vi "Image Display Loop.vi"(0 "fpga interface in":refnum<k20>, 1 "'stop' notifier":refnum<notifier>, 2 "rate references":T1(array[cluster]), 5 "raw display notifier":refnum<notifier>, 7 "display references":refnum<vi>[](array[refnum]), 11 "error in (no error)":errorcluster) -> (15 "error out":errorcluster)   [LabVIEW 2023, in "GettingStarted_Common_148X_Host.lvlib"]
uses:
  GettingStarted_Common_148X_Host.lvlib
  <vilib>/vision/Image Controls.llb/IMAQ Image.ctl
  Types/Serial Channel Display Parameters.ctl
  Types/RAW Interpretation for Display.ctl
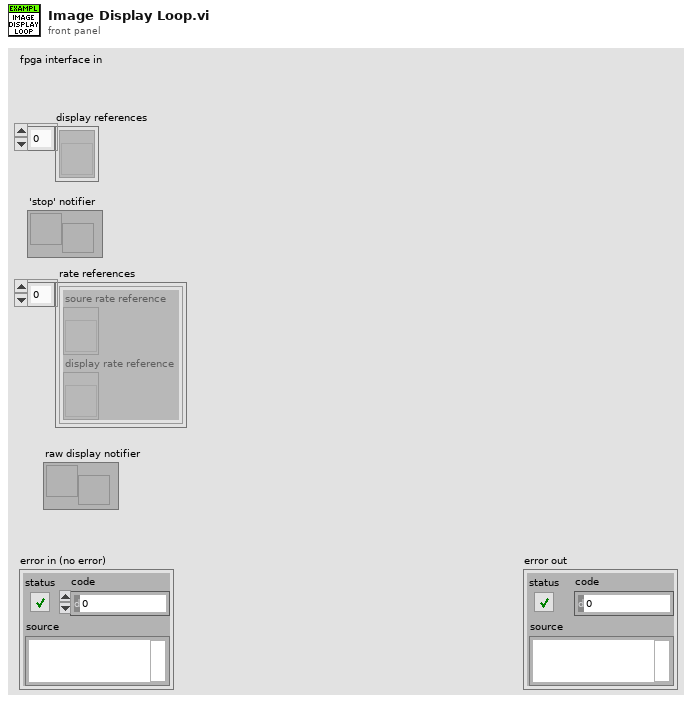
[diagram p1: front panel]
types:
  T1 = cluster{"soure rate reference":refnum<vi>, "display rate reference":refnum<vi>}[]
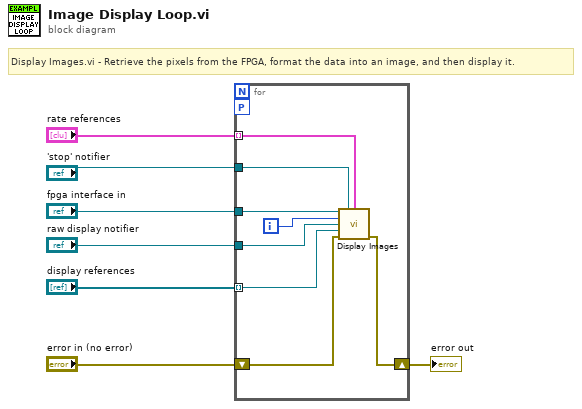
[diagram p0: block diagram]
diagram:
  # "Display Images.vi - Retrieve the pixels from the FPGA, format the data into an image, and then display it."
  n1 = for {
    tunnel: "fpga interface in" -> [w15]
    shift-right: [w12] -> w6
    shift-left: "error in (no error)" -> [w13]
    tunnel: "display references" -> [w14] mode=indexing
    tunnel: "rate references" -> [w10] mode=indexing
    workers-P: _ -> [_]
    tunnel: "'stop' notifier" -> [w9]
    tunnel: "raw display notifier" -> [w8]
    i -> [w11]
    n2 = call "Display Images.vi"("fpga interface in"=w15, "'stop' notifier"=w9, "rate references"=w10, "display channel number"=w11, "raw display notifier"=w8, "display reference"=w14, "error in (no error)"=w13) -> ("error out"=w12:errorcluster)  [unwired: 7 in, 1 out]
  }
  "error out" <- w6
